vi "Check data fits.vi"(8 "error in":errorcluster, 10 "Ext size":T1, 11 "size":u32) -> (0 "error out":errorcluster, 1 "Fits?":bool, 2 "Ext size":T1, 3 "size":u32)   [LabVIEW 2020, in "MessagePack.lvlib" / "MsgPackExt.lvclass"]
uses:
  MsgPackExt.lvclass
  Requested ext size.ctl
  <vilib>/Utility/error.llb/Error Cluster From Error Code.vi
  <vilib>/ErrorRing/Error Ring.xnode
  MsgPackExt.lvclass/MsgPackExt.ctl
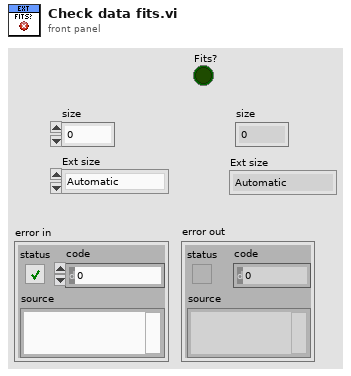
[diagram p1: front panel]
types:
  T1 = typedef "MessagePack.lvlib/MsgPackExt.lvclass/Requested ext size.ctl" = enum16{"Automatic", "Fixed 1-byte", "Fixed 2-bytes", "Fixed 4-bytes", "Fixed 8-bytes", "Fixed 16-bytes", "Up to 8 bytes", "Up to 16 bytes", "Up to 32 bytes"}
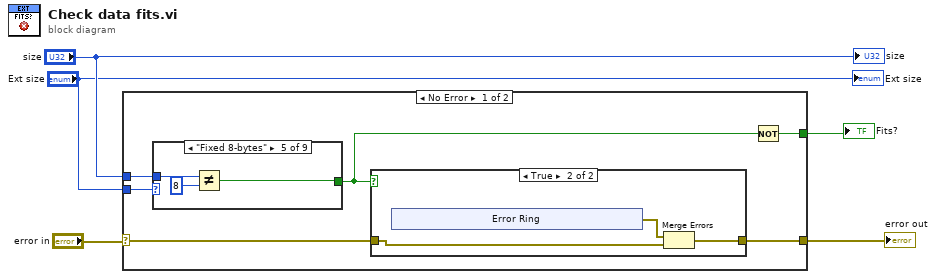
[diagram p0: block diagram]
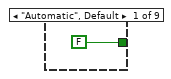
[diagram p3: hidden frame]
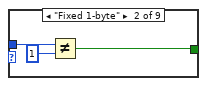
[diagram p4: hidden frame]
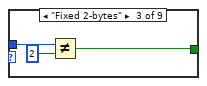
[diagram p5: hidden frame]
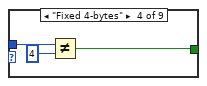
[diagram p6: hidden frame]
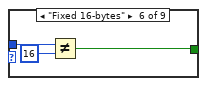
[diagram p7: hidden frame]
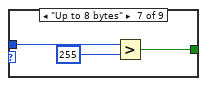
[diagram p8: hidden frame]
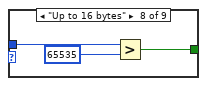
[diagram p9: hidden frame]
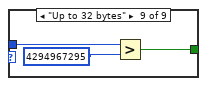
[diagram p10: hidden frame]
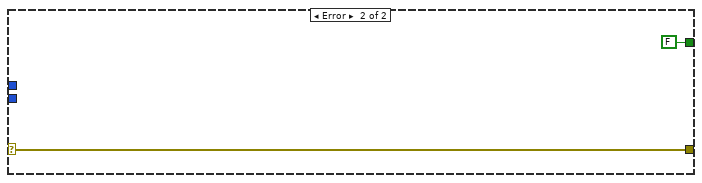
[diagram p11: hidden frame]
diagram:
  n1 = case shown="No Error" "error in" {
    selector: "error in" -> [w8 w46]
    tunnel: [w11 w46] -> w5
    tunnel: "size" -> [w10 _]
    tunnel: "Ext size" -> [w9 _]
    tunnel: [w6 FALSE] -> w1
    frame No Error {
      n2 = case shown="\"Fixed 8-bytes\"" w9 {
        tunnel: w10 -> [_ w23 w26 w29 w32 w35 w38 w41 w44]
        tunnel: [FALSE w21 w24 w27 w30 w33 w36 w39 w42] -> w7
        frame "Automatic", Default {
        }
        frame "Fixed 1-byte" {
          n3 = Not Equal?(x=w23, y=u32 1) -> (x != y?=w21:bool)
        }
        frame "Fixed 2-bytes" {
          n4 = Not Equal?(x=w26, y=u32 2) -> (x != y?=w24:bool)
        }
        frame "Fixed 4-bytes" {
          n5 = Not Equal?(x=w29, y=u32 4) -> (x != y?=w27:bool)
        }
        frame "Fixed 8-bytes" {
          n6 = Not Equal?(x=w32, y=u32 8) -> (x != y?=w30:bool)
        }
        frame "Fixed 16-bytes" {
          n7 = Not Equal?(x=w35, y=u32 16) -> (x != y?=w33:bool)
        }
        frame "Up to 8 bytes" {
          n8 = Greater?(x=w38, y=255) -> (0:w36:bool)
        }
        frame "Up to 16 bytes" {
          n9 = Greater?(x=w41, y=u32 65535) -> (0:w39:bool)
        }
        frame "Up to 32 bytes" {
          n10 = Greater?(x=w44, y=u32 4294967295) -> (0:w42:bool)
        }
      }
      n11 = case shown="True" w7 {
        tunnel: [w12 w15] -> w11
        tunnel: w8 -> [w12 w14]
        frame False {
        }
        frame True {
          n12 = xnode "Error Ring"() -> ("error out"=w13:errorcluster)
          n13 = Merge Errors(w13, w14) -> (w15:errorcluster)
        }
      }
      n14 = Not(x=w7) -> (.not. x?=w6:bool)
    }
    frame Error {
    }
  }
  "error out" <- w5
  "Fits?" <- w1
  "size" <- "size"
  "Ext size" <- "Ext size"
